vi "Table Constructor Basic DB.vi"(6 "Primary Key":string, 8 "error in (no error)":errorcluster, 9 "Table Name":string, 10 "Database":refnum<class "Database Interface.lvclass">, 11 "Table Configuration Basic DB in":refnum<class "Table Configuration Basic DB.lvclass">) -> (0 "error out":errorcluster, 3 "Table Configuration Basic DB out":refnum<class "Table Configuration Basic DB.lvclass">)   [LabVIEW 2020, in "Table.lvlib" / "Table Configuration Basic DB.lvclass"]
uses:
  Table Configuration Basic DB.lvclass
  C:/Users/User/Desktop/Raman Program/Database OOP/source/Database OOP/Table Libraries/Basic Table/Configuration/Table Configuration Class/Table Configuration.lvclass
  Database Libraries/Database Interfaces/Database Interface Class/Database Interface.lvclass
  Table Configuration Basic DB.lvclass/Table Configuration Basic DB.ctl
  Table Configuration Class/Table Configuration.lvclass/Table Configuration.ctl
  Table Configuration Class/Table Configuration.lvclass
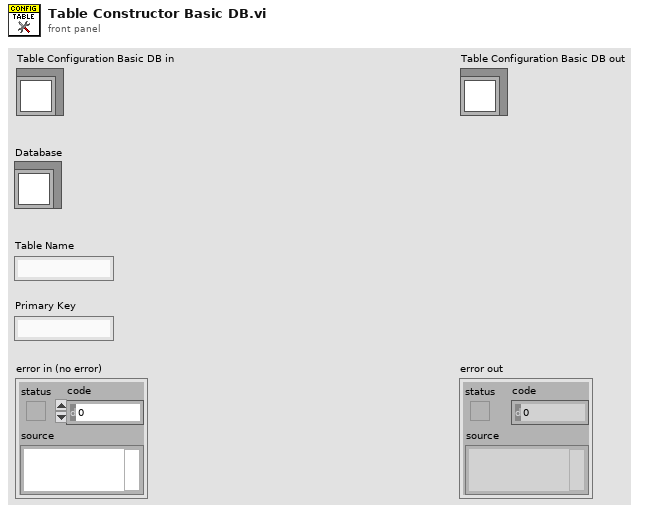
[diagram p1: front panel]
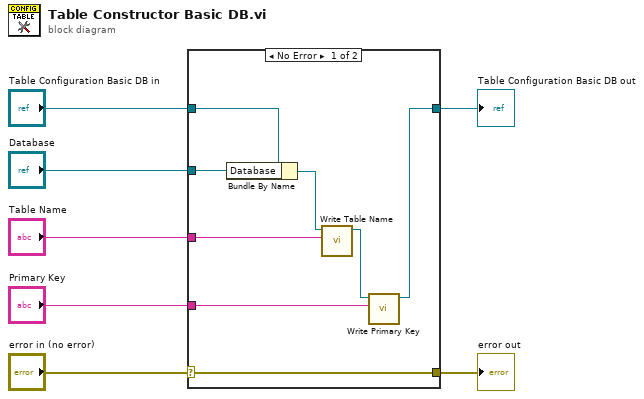
[diagram p0: block diagram]
diagram:
  n1 = case shown="No Error" "error in (no error)" {
    selector: "error in (no error)" -> [w15 w17]
    tunnel: [w15 w17] -> w6
    tunnel: [w11 w16] -> w4
    tunnel: "Table Configuration Basic DB in" -> [w14 w16]
    tunnel: "Primary Key" -> [w10 _]
    tunnel: "Table Name" -> [w9 _]
    tunnel: "Database" -> [w8 _]
    frame No Error {
      n2 = Bundle By Name(cluster=w14, "Database"=w8) -> (w13:refnum<class "Table Configuration Basic DB.lvclass">)
      n3 = call "Write Table Name.vi"("Table Name"=w9, "Table Configuration in"=w13) -> ("Table Configuration out"=w12:refnum<class "Table Configuration Basic DB.lvclass">)  [unwired: 8 in, 1 out]
      n4 = call "Write Primary Key.vi"("Primary Key"=w10, "Table Configuration in"=w12) -> ("Table Configuration out"=w11:refnum<class "Table Configuration Basic DB.lvclass">)  [unwired: 8 in, 1 out]
    }
    frame Error {
    }
  }
  "error out" <- w6
  "Table Configuration Basic DB out" <- w4
